vi "Read dInit.vi"(2 "Network Path":string, 5 "Tag Name":string) -> (1 "Numeric":i32)   [LabVIEW 2020]
uses:
  <vilib>/ethernetip/ethernetip.llb/EthernetIP Tag Read DINT.vi
  <vilib>/ethernetip/ethernetip.lvlib
panel:
  out "error out":errorcluster
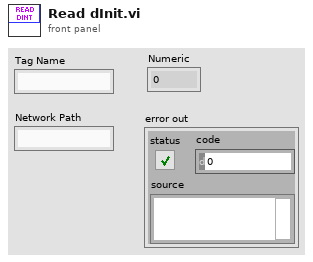
[diagram p1: front panel]
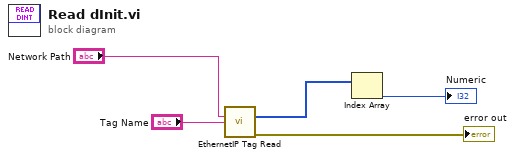
[diagram p0: block diagram]
diagram:
  n1 = call-poly <vilib>:"EthernetIP Tag Read.vi"("Network Path"="Network Path", "Tag Name"="Tag Name") -> ("Data"=w1:i32[], "error out"=→"error out":errorcluster)  [unwired: 3 in, 9 out]
  n2 = Index Array(array=w1) -> (element=→"Numeric":i32)  [unwired: 1 in]
